vi "Flatten XML String.vi"(7 "Root ID":string, 8 "Error In":errorcluster, 11 "Tree Manager":T1) -> (0 "Error Out":errorcluster, 1 "XML String":string, 3 "Tree Manager":T1)   [LabVIEW 2016, in "Tree Manager.lvclass"]
doc: "Delete Tree and all its children. \n\nIf any of the deleted Trees contained attributes of Tree Data.lvclass data type, those attributes will be realeased with the Release.vi dynamically dispatched method.\n\n<b>WARNING</b> All Tree names that contain a space character will have it replaced by underscore character. This is required by XML specification."
uses:
  Tree Manager.lvclass
  Typedefs/Session Handle.ctl
  Tree Manager.lvclass/Tree Manager.ctl
  <vilib>/xml/Close Reference(Node).vi
  <vilib>/xml/NI_XML.lvlib
  <resource>/objmgr/DOMUserDefRef.rc
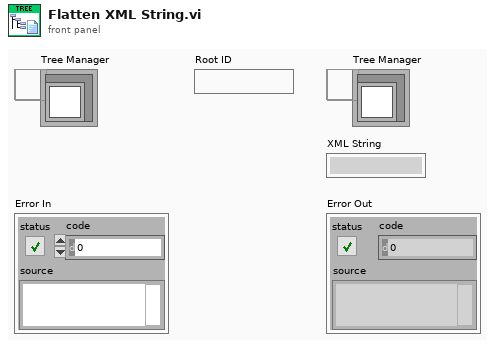
[diagram p1: front panel]
types:
  T1 = typedef "Tree Manager.lvclass/Session Handle.ctl" = refnum<data-value>
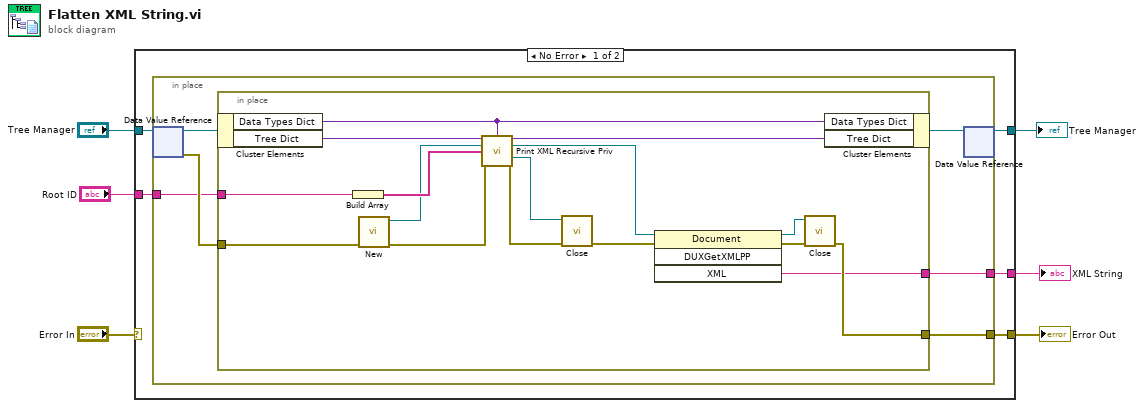
[diagram p0: block diagram]
diagram:
  n1 = case shown="No Error" "Error In" {
    selector: "Error In" -> [_ w34]
    tunnel: "Tree Manager" -> [w11 w35]
    tunnel: [w10 w35] -> w5
    tunnel: [w9 w34] -> w3
    tunnel: "Root ID" -> [w8 _]
    tunnel: [w7 _] -> w1
    frame No Error {
      n2 = in-place {
        in-place-border: [w16] -> w9
        in-place-border: w8 -> [w13]
        in-place-border: [w12] -> w7
        n3 = in-place-dvr #1(w11) -> (w17:refnum<class "Tree Manager.lvclass">, w14:errorcluster)
        n4 = in-place {
          in-place-border: [w22] -> w16
          in-place-border: w14 -> [w28]
          in-place-border: w13 -> [w31]
          in-place-border: [w21] -> w12
          n5 = in-place-cluster #2(w17) -> ("Data Types Dict"=w29:variant, "Tree Dict"=w33:variant)
          n6 = Build Array(w31) -> (w30:string[])
          n7 = call <vilib>:"New.vi"("error in (no error)"=w28) -> ("error out"=w27:errorcluster, "DOM document out"=w26:refnum<k20>)  [unwired: 7 in]
          n8 = call "Print XML Recursive Priv.vi"("Tree Dictionary In"=w33, "Data Types Dict"=w29, "DOM Doc In"=w26, "Child IDs"=w30, "error in"=w27) -> ("Tree Dictionary Out"=w32:variant, "DOM Doc Out"=w23:refnum<k20>, "Parent Node Out"=w20:refnum<k20>, "error out"=w19:errorcluster)  [unwired: 7 in]
          n9 = call-poly <vilib>:"Close.vi"("error in (no error)"=w19, "node"=w20) -> ("error out"=w18:errorcluster)  [unwired: 7 in]
          n10 = invoke class="Document" method="DUXGetXMLPP"(reference=w23, error in=w18) -> (reference out=w24:refnum<k20>, error out=w25:errorcluster, "XML"=w21:string)  [unwired: 2 in, 1 out]
          n11 = call-poly <vilib>:"Close.vi"("error in (no error)"=w25, "node"=w24) -> ("error out"=w22:errorcluster)  [unwired: 7 in]
          n12 = in-place-cluster #2("Data Types Dict"=w29, "Tree Dict"=w32) -> (w15:refnum<class "Tree Manager.lvclass">)
        }
        n13 = in-place-dvr #1(w15) -> (w10:T1)  [unwired: 1 out]
      }
    }
    frame Error {
    }
  }
  "Tree Manager" <- w5
  "Error Out" <- w3
  "XML String" <- w1
